vi "OdorSystem-counter-V1.vi"() -> ()   [LabVIEW 2019]
doc: "Synchronize Correlated Digital Output with Analog Input Using NI-DAQmx \n\nOverview:\nThis example uses DAQmx to synchronize finite generation and acquisition of Correlated Digital Output with an Analog Input Task respectively.\n\nDescriptions:\nCorrelated I/O enables synchronization of on board digital I/O lines to a clock reference. Digital and Analog samples can be synchronized in time by sharing the AI clock as the source of your digital I/O clock. You may also use the Counter Output pulse as the Source of Digital Timing. Hence, set the Source for Digital Timing as ai/SampleClock.This example will work on any device that uses DAQmx and supports Correlated Digital I/O. To perform Correlated Digital I/O on 9172 Chassis, you need a Correlated Module in slot 1-4 of the chassis. \n\nRequirements:\n1. LabVIEW 2012 or compatible.\n2. NI-DAQmx 15.5.1 or compatible.\n\nInstructions:\n1. Set all the control values on the front panel corresponding to the physical channel to be used on the DAQ device.\n2. Run this VI.\n3. Monitor the analog input voltage measured and ramp signal generated from specified channels. \n\nBlock Diagram Steps:\n1. Creates channels to measure voltage and to generate digital signals \n2. Sets the source of the Sample Clock, the rate of the Sample Clock, and the number of samples to acquire or generate.\n3. Generates an array containing a ramp pattern and write to digital output lines.\n4. Transitions the tasks to running state to begin measuring and generating data.\n5. Reads the waveform from the analog input channel and waits for the digital output generation to complete.\n6. Clears the tasks.\n7. Displays any error occurs."
uses:
  StatesEnum.ctl
  <vilib>/DAQmx/write.llb/DAQmx Write (Digital 1D Bool NChan 1Samp 1Line).vi
  <vilib>/DAQmx/write.llb/DAQmx Write (Digital Wfm 1Chan NSamp).vi
  <vilib>/DAQmx/miscellaneous.llb/DAQmx Fill In Error Info.vi
  <vilib>/DAQmx/create/channels.llb/DAQmx Create Channel (CO-Pulse Generation-Frequency).vi
  <vilib>/Waveform/DWDTOps.llb/Digital Pattern Generator (Single Value).vi
  <vilib>/Waveform/DWDTOps.llb/DWDT Append Digital Samples.vi
  <vilib>/DAQmx/configure/timing.llb/DAQmx Timing (Implicit).vi
  <vilib>/Waveform/DWDTOps.llb/DWDT Append Digital Signals.vi
  <vilib>/Waveform/DWDTOps.llb/DWDT Digital to Boolean Array.vi
  <vilib>/DAQmx/create/channels.llb/DAQmx Create Channel (DO-Digital Output).vi
  <vilib>/DAQmx/configure/timing.llb/DAQmx Timing (Sample Clock).vi
  <vilib>/Waveform/DWDTOps.llb/DWDT Uncompress Digital.vi
panel:
  out "Experiment running":bool
  out "State":T1
  in  "Select experiment":enum32{"Single trial", "Trial series"}(tab)
  out "Time elapsed":dbl format="%.1f"
  in  "Start single trial":bool
  out "single trial done":bool
  in  "Select valve":u8(knob)=1 min=1 max=8 step=1 scale=1.0..8.0
  out "Pause elapsed time":dbl format="%#.1f"
  out "In between trials":bool
  out "Trial elapsed time":dbl format="%.1f"
  out "Total elapsed time":dbl format="%.1f"
  out "Estimated total time":dbl
  out "Current list index":i32
  out "Current Valve":u8
  in  "Time between trials":u16=10 min=1 max=900 step=1
  in  "Start trial series":bool
  in  "Valve order list":i8[](array[numeric]) min=1 max=8 step=1
  out "Digitaler output":digitalwaveform(graph)
  out "Stop Boolesch":bool
  in  "Total trial time":dbl=20.0 min=1.0 step=0.1
  in  "Valve opening Time":dbl=10.0 min=0.0 step=0.1
  in  "Valve delay":dbl=2.0 min=0.0 step=0.1
  in  "Stopp":bool
  out "Digital Waveform Graph":digitalwaveform(graph)
  # "All times are in second!"
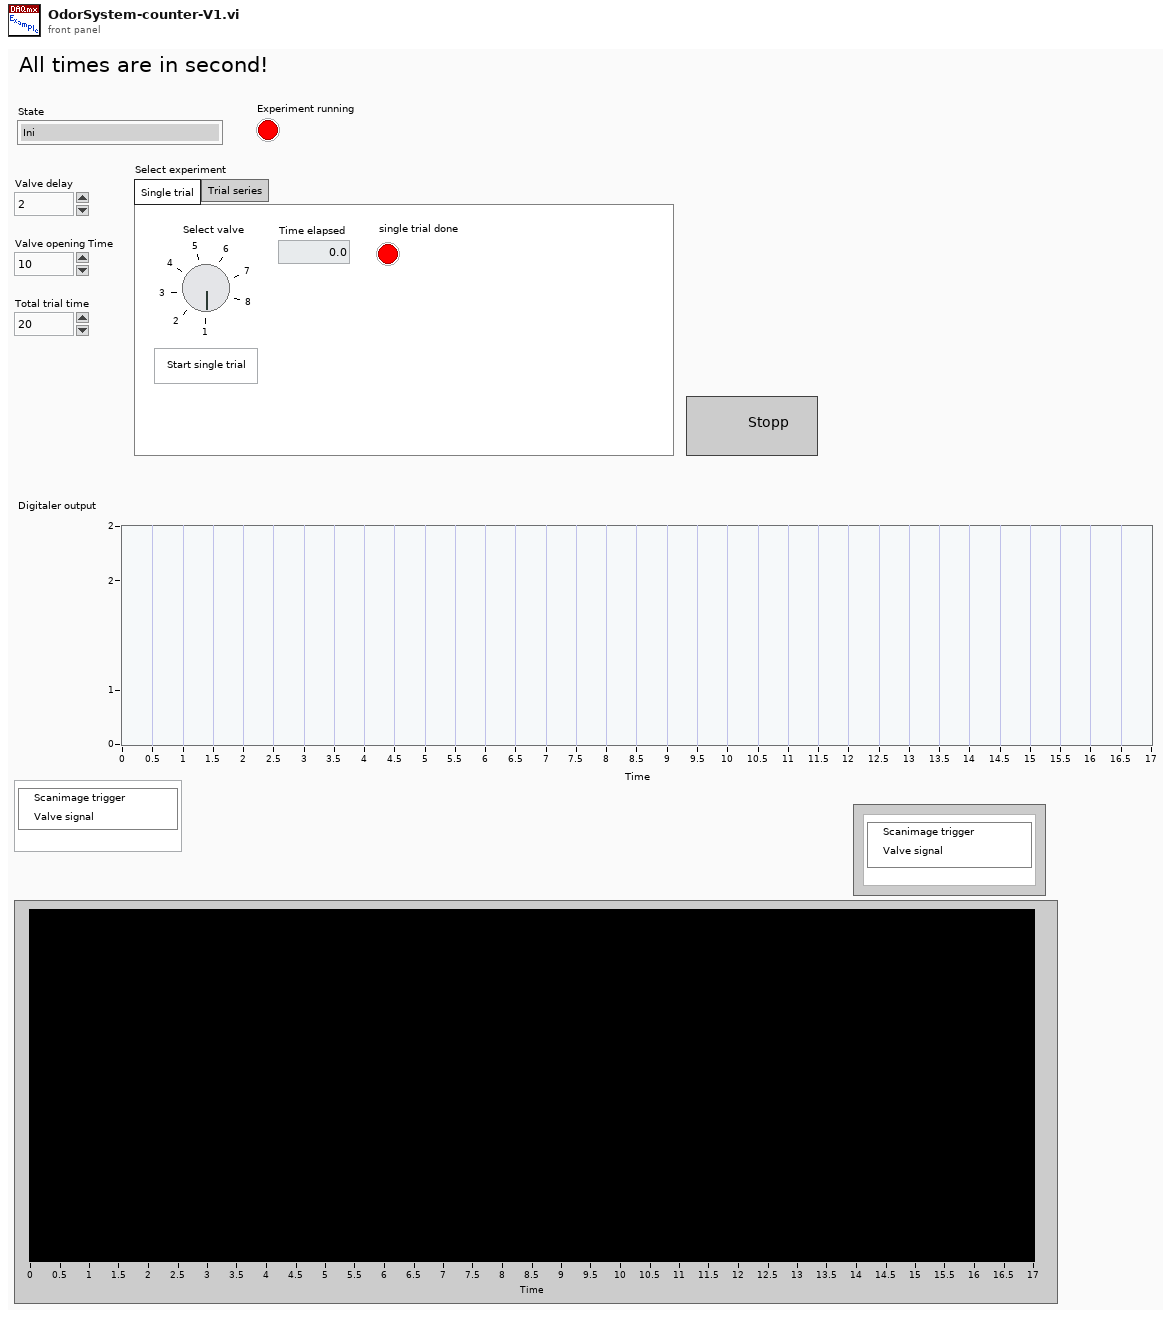
[diagram p1: front panel]
types:
  T1 = typedef "StatesEnum.ctl" = enum16{"Ini", "Standby", "Start Trial", "Start trial series", "Stop"}
  T2 = enum8{"Enabled", "Disabled", "Disabled and Grayed Out"}
  T3 = enum32{"Page Enabled", "Page Disabled", "Page Disabled & Grayed"}
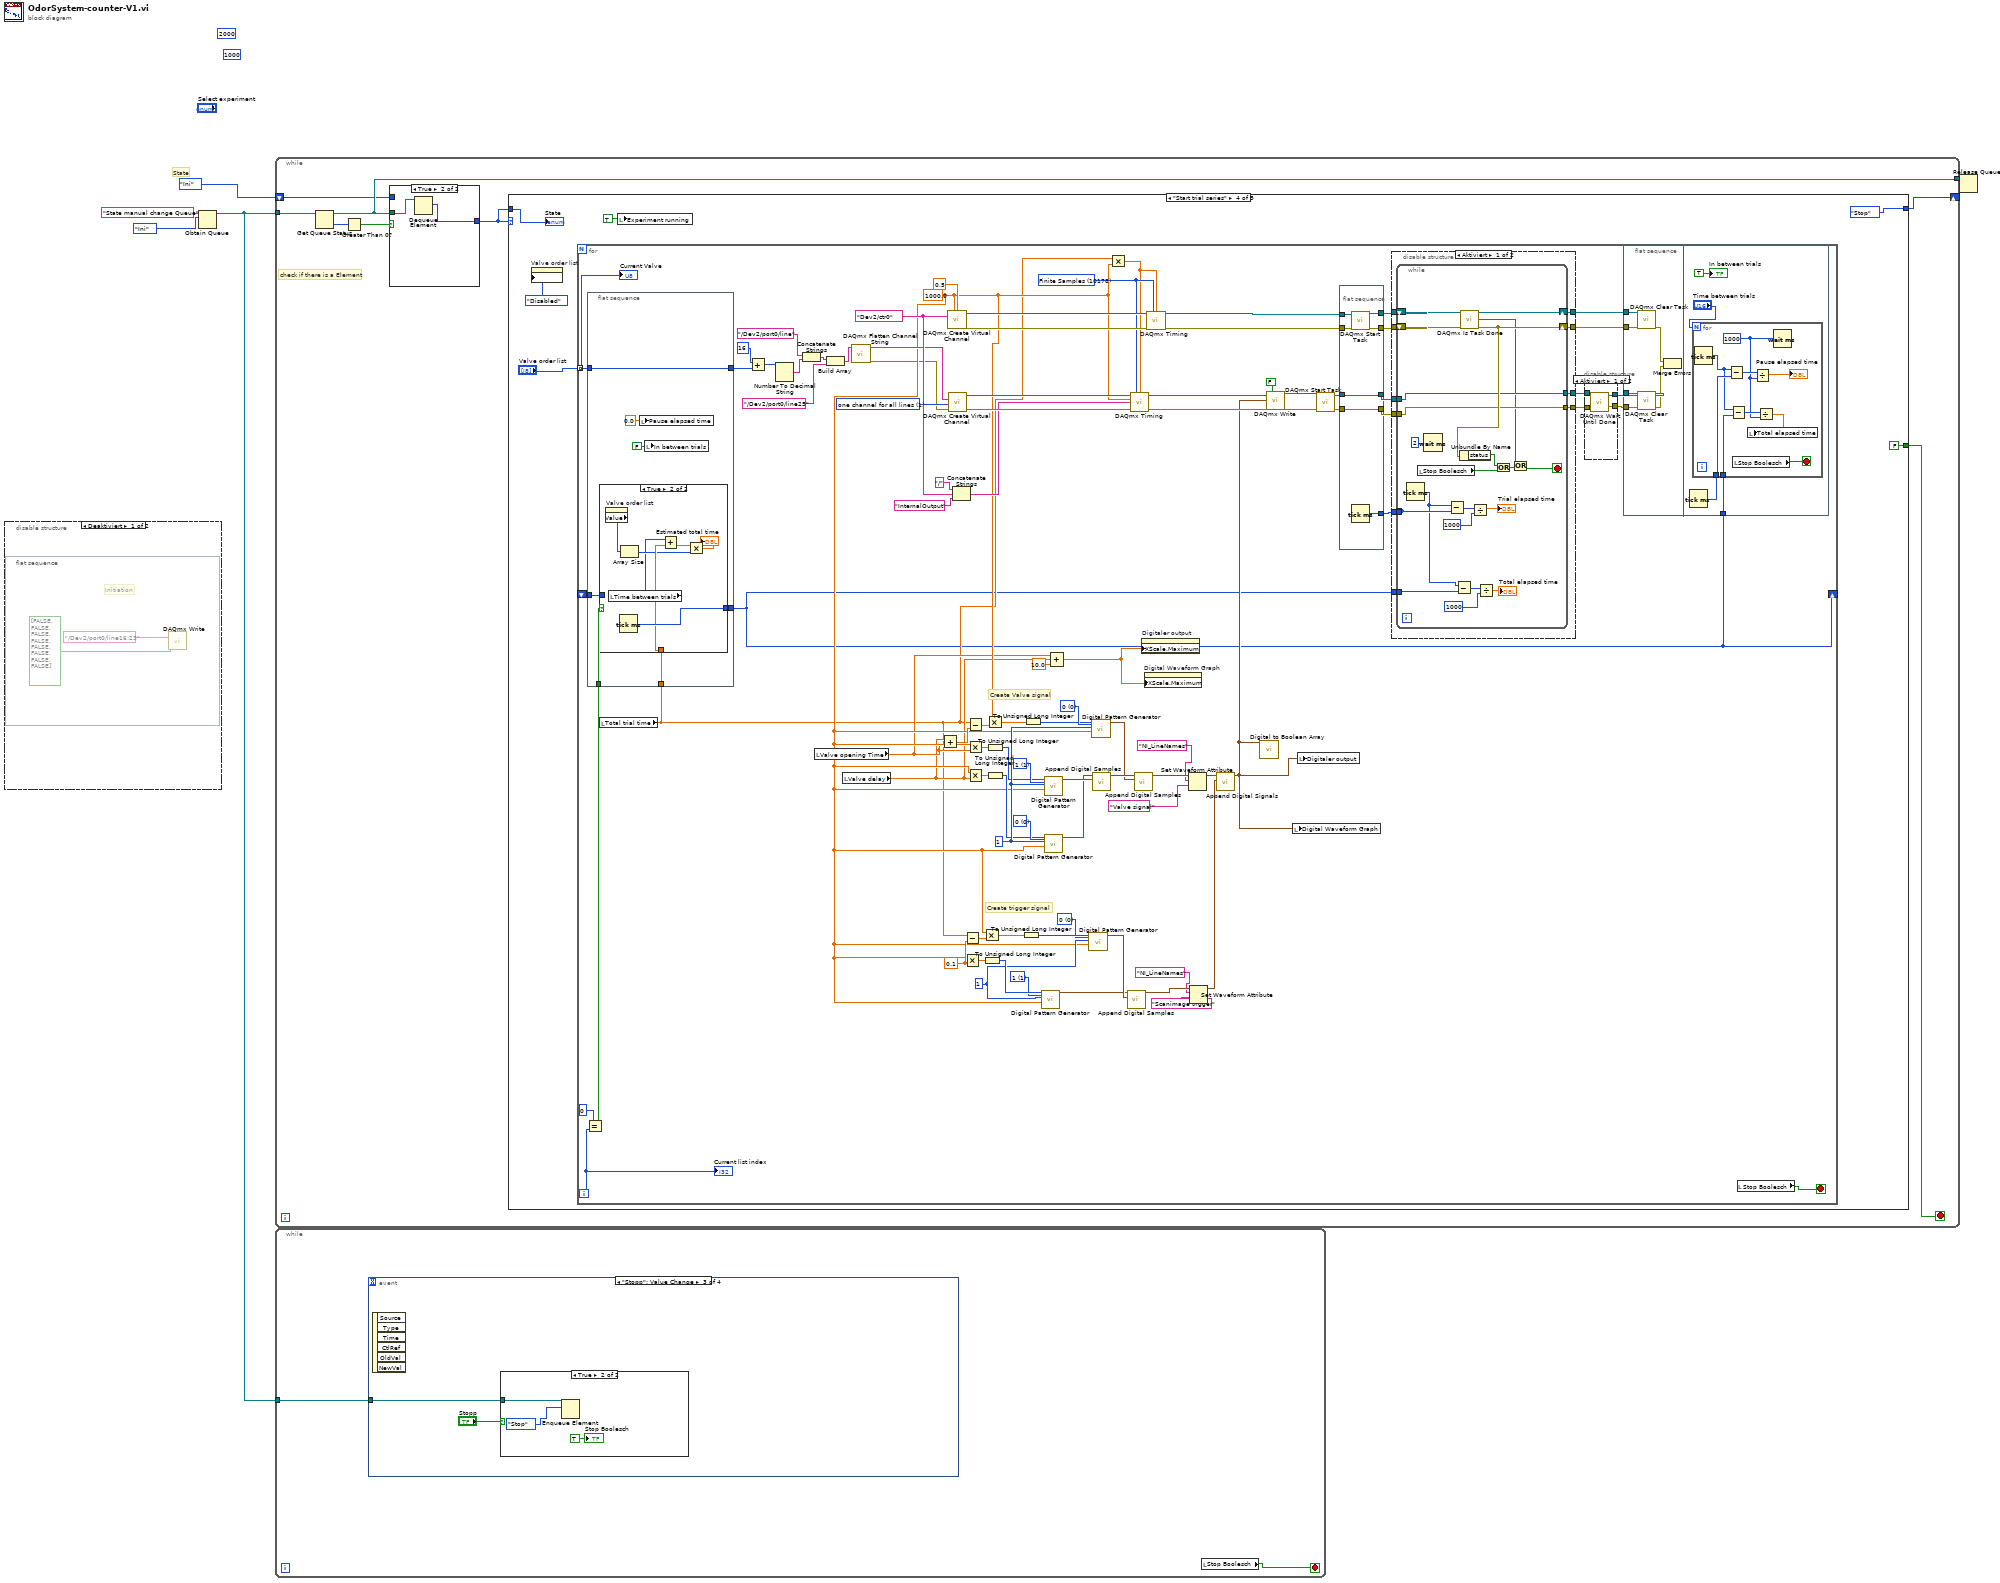
[diagram p0: block diagram]
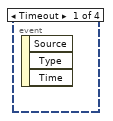
[diagram p3: hidden frame]
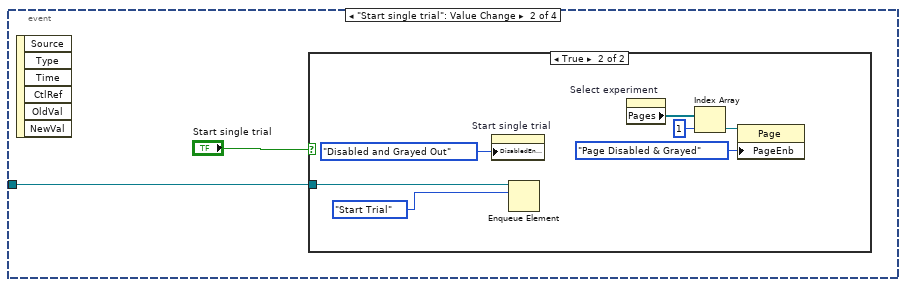
[diagram p4: hidden frame]
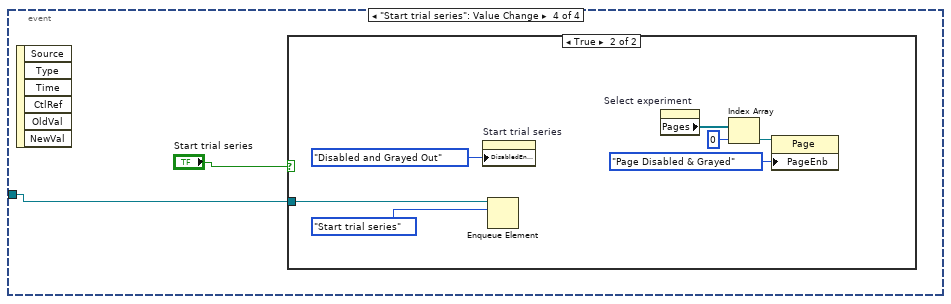
[diagram p7: hidden frame]
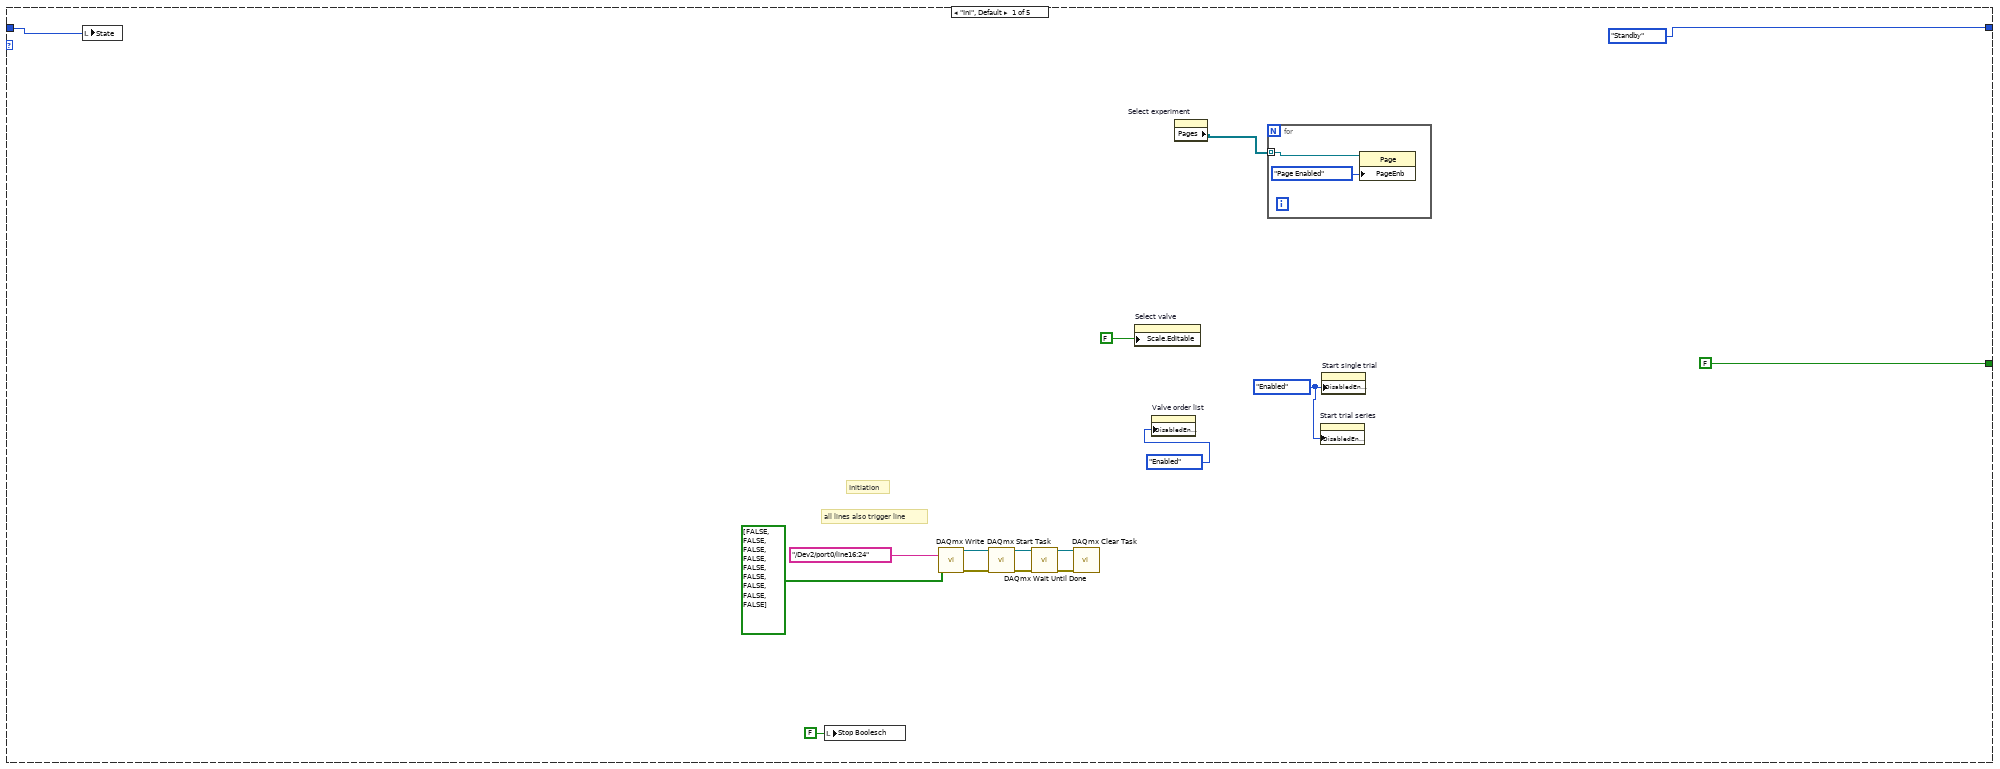
[diagram p10: hidden frame]
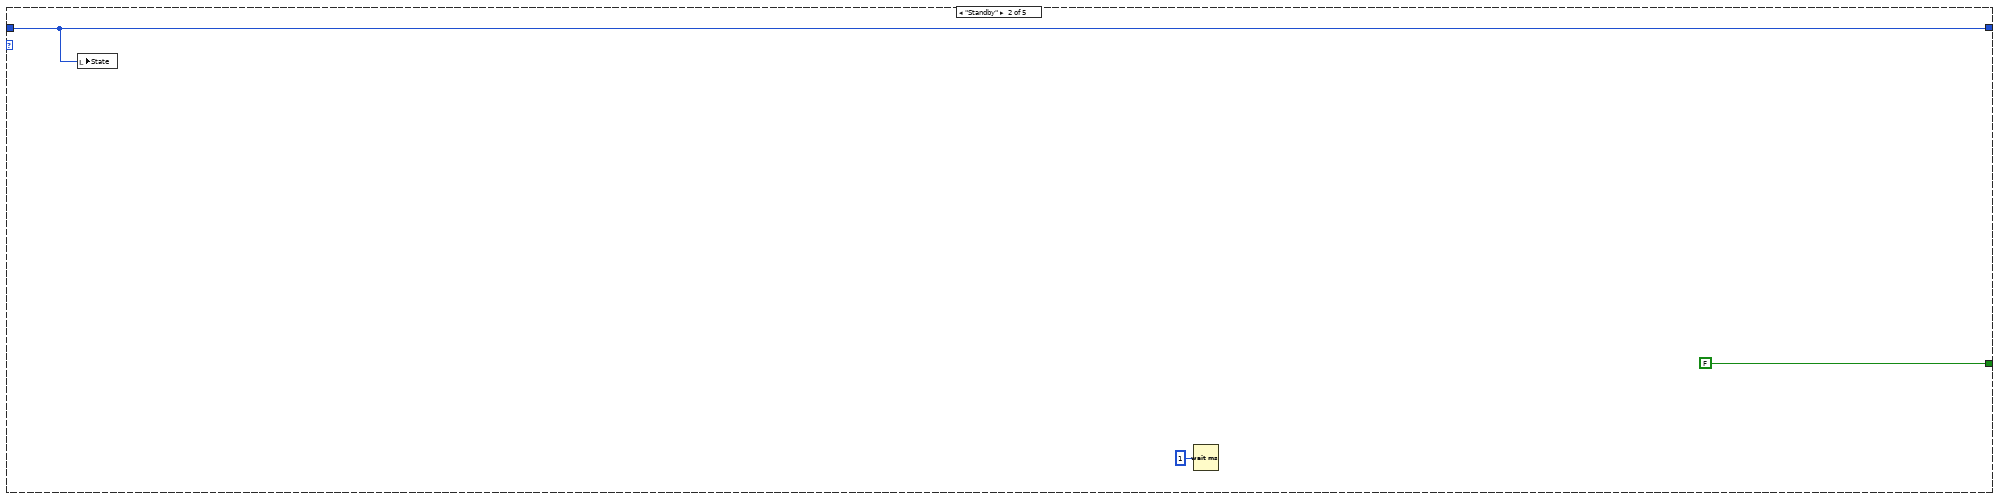
[diagram p11: hidden frame]
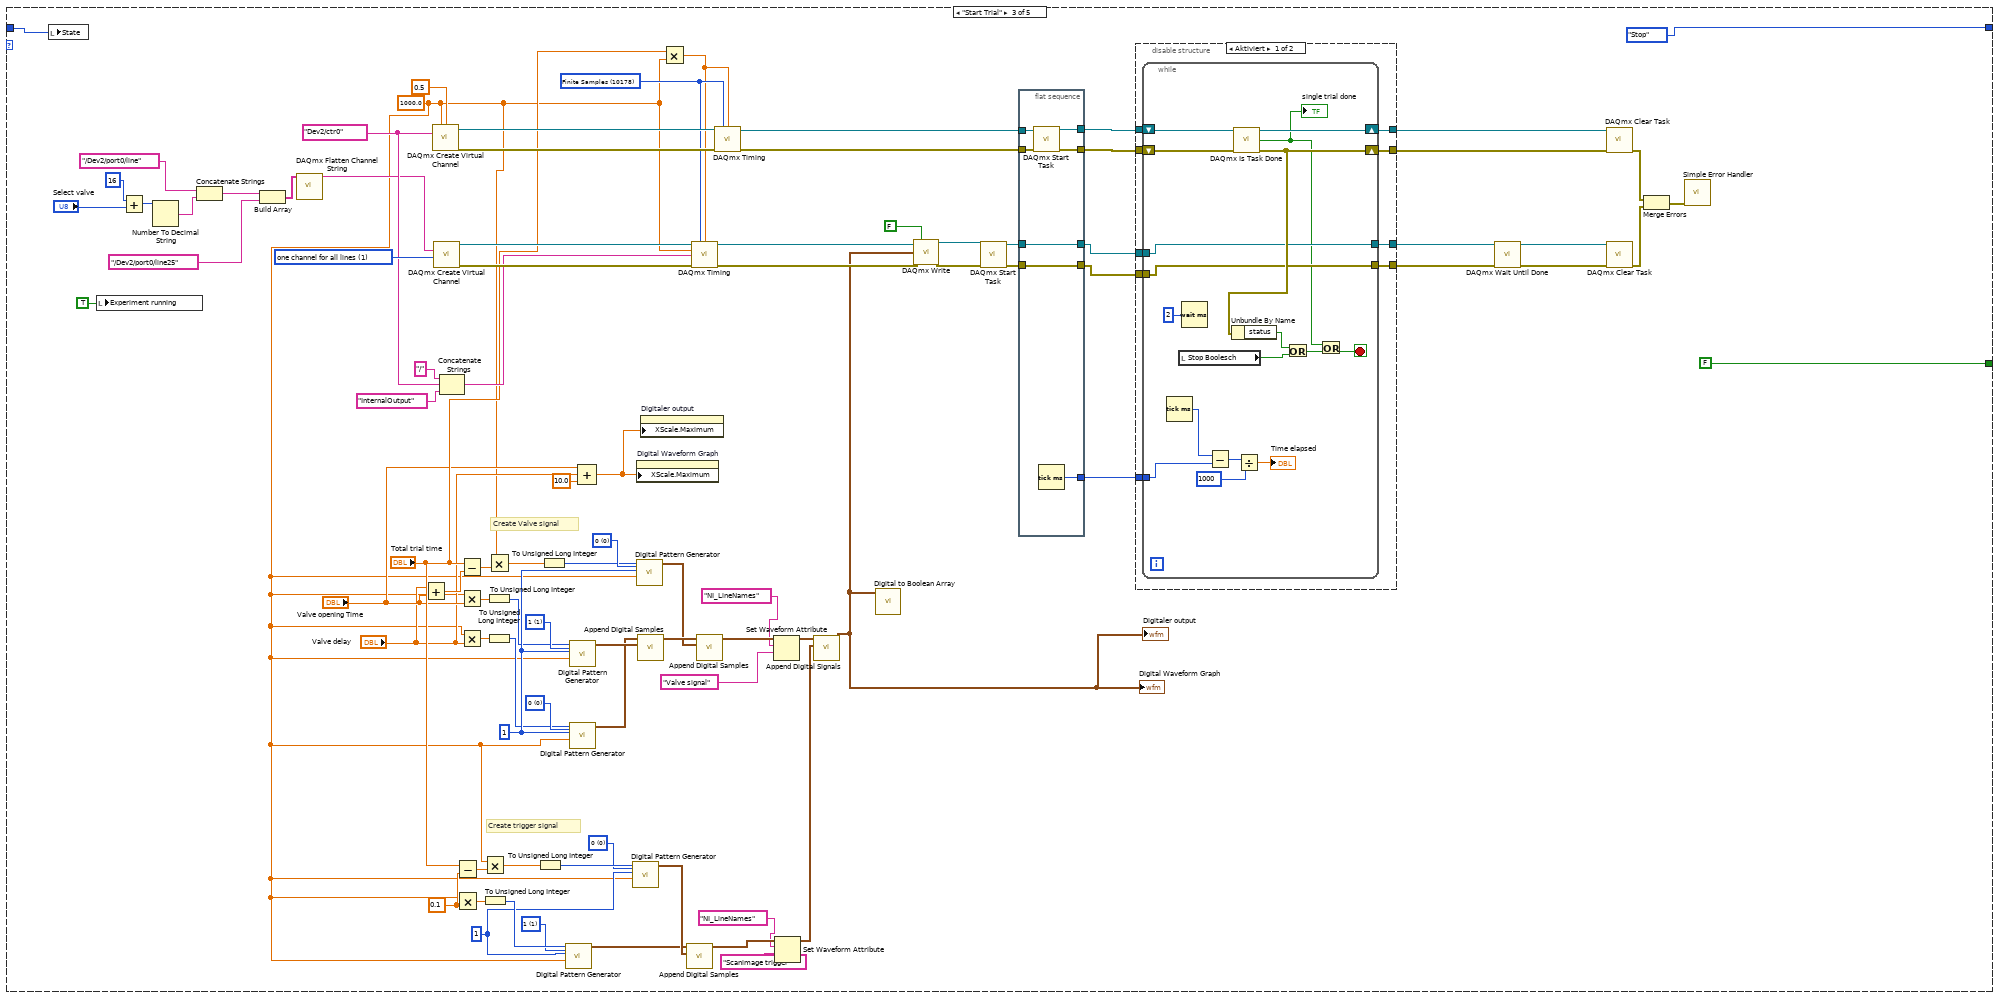
[diagram p12: hidden frame]
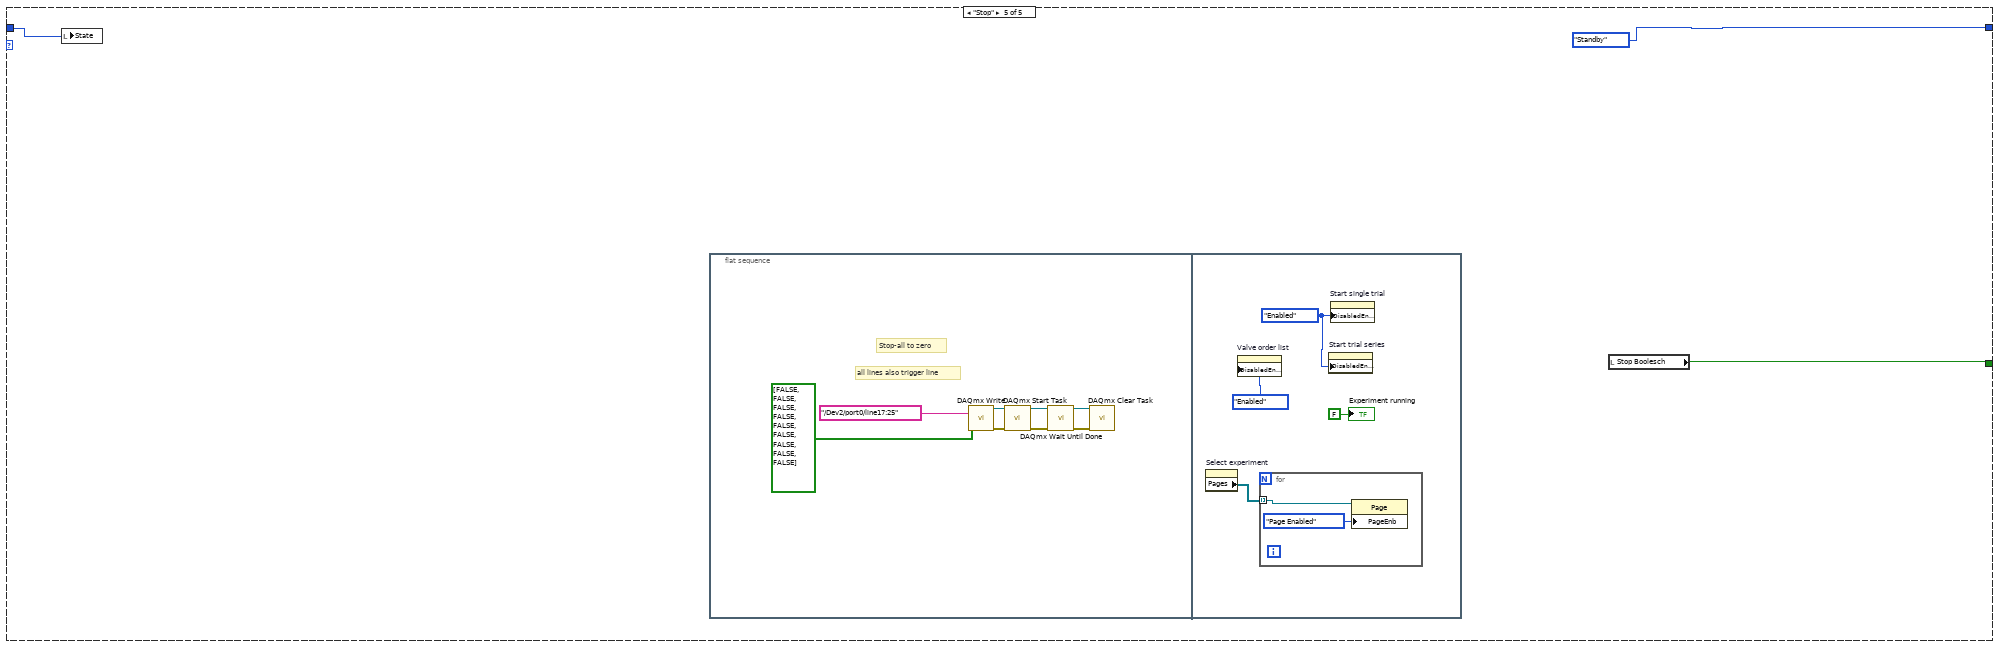
[diagram p17: hidden frame]
diagram:
  (unwired) u32 2000 ("number of samples")
  (unwired) u32 1000 ("number of samples")
  # "State"
  n1 = disable-structure shown="Deaktiviert" {
    frame Disabled {
      n2 = flat-sequence {
        frame #0 {
          # "Initiation"
          n3 = call-poly <vilib>:"DAQmx Write.vi"("task/channels in"="/Dev2/port0/line16:23" ("string"), "data"=bool[] [FALSE, FALSE, FALSE, FALSE, FALSE, FALSE, FALSE, FALSE]) -> ()  [unwired: 11 in, 3 out]
        }
      }
    }
    frame Enabled {
    }
  }
  n4 = Obtain Queue(name (unnamed)="State manual change Queue", element data type=StatesEnum."Ini" ("Enum")) -> (queue out=w4:refnum<queue>)  [unwired: 3 in, 2 out]
  n5 = while {
    tunnel: w4 -> [w13]
    tunnel: [w12] -> w3
    shift-right: [w8] -> _
    shift-left: StatesEnum."Ini" -> [w9]
    stop <- w11 stop-if-true
    # "check if there is a Element"
    n6 = Get Queue Status(queue=w13) -> (queue out=w12:refnum<queue>, # elements in queue=w15:i32)  [unwired: 2 in, 6 out]
    n7 = Greater Than 0?(x=w15) -> (x > 0?=w14:bool)
    n8 = case shown="True" w14 {
      tunnel: w12 -> [_ w18]
      tunnel: w9 -> [w16 _]
      tunnel: [w16 w17] -> w10
      frame False {
      }
      frame True {
        n9 = Dequeue Element(queue=w18) -> (element=w17:T1)  [unwired: 2 in, 3 out]
      }
    }
    n10 = case shown="\"Start trial series\"" w10 {
      tunnel: w10 -> [w29 w37 w43 w165 w335]
      tunnel: [FALSE ("Stop Boolesch") FALSE ("Stop Boolesch") FALSE ("Stop Boolesch") FALSE ("Stop Boolesch") w337] -> w11
      tunnel: [StatesEnum."Standby" ("Enum") w37 StatesEnum."Stop" ("Enum") StatesEnum."Stop" ("Enum") StatesEnum."Standby" ("Enum")] -> w8
      frame "Ini", Default {
        w22 = T2."Enabled" ("Deaktiviert")
        # "all lines also trigger line"
        # "Initiation"
        n11 = local write "State"(w29) -> ()
        n12 = local write "Stop Boolesch"(FALSE ("Stop Boolesch")) -> ()
        n13 = call-poly <vilib>:"DAQmx Write.vi"("task/channels in"="/Dev2/port0/line16:24" ("string"), "data"=bool[] [FALSE, FALSE, FALSE, FALSE, FALSE, FALSE, FALSE, FALSE, FALSE]) -> ("task out"=w24:refnum<k21>, "error out"=w23:errorcluster)  [unwired: 11 in, 1 out]
        n14 = call <vilib>:"DAQmx Start Task.vi"("task/channels in"=w24, "error in"=w23) -> ("task out"=w28:refnum<k21>, "error out"=w26:errorcluster)  [unwired: 12 in]
        n15 = call <vilib>:"DAQmx Wait Until Done.vi"("task/channels in"=w28, "error in"=w26) -> ("task out"=w27:refnum<k21>, "error out"=w25:errorcluster)  [unwired: 12 in]
        n16 = call <vilib>:"DAQmx Clear Task.vi"("task in"=w27, "error in"=w25) -> ()  [unwired: 13 in, 1 out]
        n17 = property on="Select valve" class="Knob (strict)"("Scale.Editable"=FALSE ("Skala.Editierbar")) -> ()  [unwired: 2 in, 2 out]
        n18 = property on="Valve order list" class="Arr (strict)"("DisabledEnum"=T2."Enabled" ("Deaktiviert")) -> ()  [unwired: 2 in, 2 out]
        n19 = property on="Select experiment" class="TabCtl (strict)"() -> ("Pages"=w20:refnum<vi>[])  [unwired: 2 in, 2 out]
        n20 = for {
          tunnel: w20 -> [w35] mode=indexing
          n21 = property class="Page"(reference=w35, "PageEnb"=T3."Page Enabled" ("Aktiv-Status der Seite")) -> ()  [unwired: 1 in, 2 out]
        }
        n22 = property on="Start trial series" class="Bool"("DisabledEnum"=w22) -> ()  [unwired: 2 in, 2 out]
        n23 = property on="Start single trial" class="Bool"("DisabledEnum"=w22) -> ()  [unwired: 2 in, 2 out]
      }
      frame "Standby" {
        n24 = local write "State"(w37) -> ()
        n25 = Wait (ms)(milliseconds to wait=u32 1 ("Zu wartende ms")) -> ()  [unwired: 1 out]
      }
      frame "Start Trial" {
        w67 = 0.1 ("y")
        w74 = u32 1 ("number of signals")
        w76 = u8 0 items=["0", "1", "Z", "L", "H", "X", "T", "V"] ("value")
        w75 = u8 1 items=["0", "1", "Z", "L", "H", "X", "T", "V"] ("value")
        w95 = tag "Dev2/ctr0" ("counter")
        w49 = 1000.0 ("frequency")
        w104 = u32 1 ("number of signals")
        w105 = u8 0 items=["0", "1", "Z", "L", "H", "X", "T", "V"] ("value")
        w106 = u8 1 items=["0", "1", "Z", "L", "H", "X", "T", "V"] ("value")
        w107 = u8 0 items=["0", "1", "Z", "L", "H", "X", "T", "V"] ("value")
        w118 = 1 items=["one channel for each line", "one channel for all lines"] ("line grouping")
        w99 = 10178 items=["Finite Samples"=10178, "Continuous Samples"=10123] ("sample mode")
        # "Create trigger signal"
        # "Create Valve signal"
        n26 = local write "State"(w43) -> ()
        n27 = local write "Experiment running"(TRUE ("Experiment running")) -> ()
        n28 = Add(x=i8 16, y="Select valve") -> (x+y=w83:u8)
        n29 = Number To Decimal String(number=w83) -> (decimal integer string=w84:string)  [unwired: 1 in]
        n30 = Concatenate Strings("/Dev2/port0/line" ("string"), w84) -> (w73:string)
        n31 = Build Array(w73, "/Dev2/port0/line25" ("string")) -> (w71:string[])
        n32 = call <vilib>:"DAQmx Flatten Channel String.vi"("names in"=w71) -> ("names out"=w70:string)  [unwired: 13 in, 1 out]
        n33 = Add(x="Valve delay", y="Valve opening Time") -> (x+y=w87:dbl)
        n34 = call-poly <vilib>:"DAQmx Create Virtual Channel.vi"("frequency"=w49, "duty cycle"=0.5, "counter"=w95) -> ("task out"=w123:refnum<k21>, "error out"=w124:errorcluster)  [unwired: 11 in]
        n35 = call-poly <vilib>:"DAQmx Create Virtual Channel.vi"("lines"=w70, "line grouping"=w118) -> ("task out"=w128:refnum<k21>, "error out"=w127:errorcluster)  [unwired: 12 in]
        n36 = Concatenate Strings("/", w95, "InternalOutput" ("string")) -> (w94:string)
        n37 = Subtract(x="Total trial time", y=w67) -> (x-y=w81:dbl)
        n38 = Multiply(x=w49, y=w67) -> (x*y=w77:dbl)
        n39 = Subtract(x="Total trial time", y=w87) -> (x-y=w86:dbl)
        n40 = Multiply(x=w49, y="Valve opening Time") -> (x*y=w91:dbl)
        n41 = Multiply(x=w49, y="Valve delay") -> (x*y=w93:dbl)
        n42 = Multiply(x=w49, y=w81) -> (x*y=w79:dbl)
        n43 = To Unsigned Long Integer(number=w77) -> (unsigned 32bit integer=w78:u32)
        n44 = Multiply(x=w49, y=w86) -> (x*y=w89:dbl)
        n45 = To Unsigned Long Integer(number=w91) -> (unsigned 32bit integer=w90:u32)
        n46 = To Unsigned Long Integer(number=w93) -> (unsigned 32bit integer=w92:u32)
        n47 = To Unsigned Long Integer(number=w79) -> (unsigned 32bit integer=w80:u32)
        n48 = To Unsigned Long Integer(number=w89) -> (unsigned 32bit integer=w88:u32)
        n49 = call-poly <vilib>:"Digital Pattern Generator.vi"("value"=w75, "sample rate"=w49, "number of signals"=w74, "number of samples"=w78) -> ("digital waveform"=w55:digitalwaveform)  [unwired: 6 in, 1 out]
        n50 = call-poly <vilib>:"Digital Pattern Generator.vi"("value"=w106, "sample rate"=w49, "number of signals"=w104, "number of samples"=w90) -> ("digital waveform"=w60:digitalwaveform)  [unwired: 6 in, 1 out]
        n51 = call-poly <vilib>:"Digital Pattern Generator.vi"("value"=w107, "sample rate"=w49, "number of signals"=w104, "number of samples"=w92) -> ("digital waveform"=w59:digitalwaveform)  [unwired: 6 in, 1 out]
        n52 = Compound Arithmetic op=ADD("Valve opening Time", "Valve delay", 10.0 ("Wert")) -> (w44:dbl)
        n53 = call-poly <vilib>:"Digital Pattern Generator.vi"("value"=w76, "sample rate"=w49, "number of signals"=w74, "number of samples"=w80) -> ("digital waveform"=w56:digitalwaveform)  [unwired: 6 in, 1 out]
        n54 = property on="Digital Waveform Graph" class="DigitalGraph (strict)"("XScale.Maximum"=w44) -> ()  [unwired: 2 in, 2 out]
        n55 = call-poly <vilib>:"Digital Pattern Generator.vi"("value"=w105, "sample rate"=w49, "number of signals"=w104, "number of samples"=w88) -> ("digital waveform"=w57:digitalwaveform)  [unwired: 6 in, 1 out]
        n56 = call-poly <vilib>:"Append Digital Samples.vi"("digital waveform B"=w60, "digital waveform A"=w59) -> ("digital waveform out"=w58:digitalwaveform)  [unwired: 8 in, 1 out]
        n57 = property on="Digitaler output" class="DigitalGraph (strict)"("XScale.Maximum"=w44) -> ()  [unwired: 2 in, 2 out]
        n58 = Multiply(x="Total trial time", y=w49) -> (x*y=w68:dbl)
        n59 = call-poly <vilib>:"Append Digital Samples.vi"("digital waveform B"=w56, "digital waveform A"=w55) -> ("digital waveform out"=w66:digitalwaveform)  [unwired: 8 in, 1 out]
        n60 = call-poly <vilib>:"DAQmx Timing.vi"("task/channels in"=w128, "sample mode"=w99, "samples per channel"=w68, "rate"=w49, "source"=w94, "error in"=w127) -> ("task out"=w115:refnum<k21>, "error out"=w114:errorcluster)  [unwired: 8 in]
        n61 = call-poly <vilib>:"Append Digital Samples.vi"("digital waveform B"=w57, "digital waveform A"=w58) -> ("digital waveform out"=w63:digitalwaveform)  [unwired: 8 in, 1 out]
        n62 = call-poly <vilib>:"DAQmx Timing.vi"("task/channels in"=w123, "sample mode"=w99, "samples per channel"=w68, "error in"=w124) -> ("task out"=w121:refnum<k21>, "error out"=w122:errorcluster)  [unwired: 10 in]
        n63 = Set Waveform Attribute(5:"Valve signal", 6:"NI_LineNames" ("name"), 7:w63) -> (3:w54:digitalwaveform)  [unwired: 1 in, 2 out]
        n64 = Set Waveform Attribute(5:"Scanimage trigger", 6:"NI_LineNames" ("name"), 7:w66) -> (3:w53:digitalwaveform)  [unwired: 1 in, 2 out]
        n65 = call-poly <vilib>:"Append Digital Signals.vi"("digital waveform (low bits)"=w53, "digital waveform (high bits)"=w54) -> ("digital waveform out"=w46:digitalwaveform)  [unwired: 8 in, 1 out]
        "Digital Waveform Graph" <- w46
        "Digitaler output" <- w46
        n66 = call-poly <vilib>:"Digital to Boolean Array.vi"("digital waveform"=w46) -> ()  [unwired: 9 in, 2 out]
        n67 = call-poly <vilib>:"DAQmx Write.vi"("task/channels in"=w115, "auto start"=FALSE, "data"=w46, "error in"=w114) -> ("task out"=w113:refnum<k21>, "error out"=w112:errorcluster)  [unwired: 9 in, 1 out]
        n68 = call <vilib>:"DAQmx Start Task.vi"("task/channels in"=w113, "error in"=w112) -> ("task out"=w117:refnum<k21>, "error out"=w116:errorcluster)  [unwired: 12 in]
        n69 = flat-sequence {
          tunnel: [w161] -> w126
          tunnel: [w160] -> w125
          tunnel: w122 -> [w159]
          tunnel: w121 -> [w158]
          tunnel: [w157] -> w103
          tunnel: w117 -> [w157]
          tunnel: [w156] -> w102
          tunnel: w116 -> [w156]
          tunnel: [w155] -> w41
          frame #0 {
            n70 = call <vilib>:"DAQmx Start Task.vi"("task/channels in"=w158, "error in"=w159) -> ("task out"=w161:refnum<k21>, "error out"=w160:errorcluster)  [unwired: 12 in]
            n71 = Tick Count (ms)() -> (millisecond timer value=w155:u32)
          }
        }
        n72 = disable-structure shown="Aktiviert" {
          disable-tunnel: w126 -> [w137 _]
          disable-tunnel: w125 -> [w136 _]
          disable-tunnel: [w135 _] -> w120
          disable-tunnel: [w134 _] -> w119
          disable-tunnel: w103 -> [w133 _]
          disable-tunnel: w102 -> [w132 _]
          disable-tunnel: [w131 _] -> w101
          disable-tunnel: [w130 _] -> w100
          disable-tunnel: w41 -> [w129 _]
          frame Enabled {
            n73 = while {
              shift-right: [w151] -> w134
              shift-left: w137 -> [w153]
              shift-right: [w150] -> w135
              shift-left: w136 -> [w152]
              tunnel: w133 -> [w149]
              tunnel: w132 -> [w148]
              tunnel: [w149] -> w131
              tunnel: [w148] -> w130
              tunnel: w129 -> [w141]
              stop <- w144 stop-if-true
              n74 = Tick Count (ms)() -> (millisecond timer value=w142:u32)
              n75 = local read "Stop Boolesch"() -> (w145:bool)
              n76 = Wait (ms)(milliseconds to wait=u32 2 ("Zu wartende ms")) -> ()  [unwired: 1 out]
              n77 = Subtract(x=w142, y=w141) -> (x-y=w140:u32)
              n78 = call <vilib>:"DAQmx Is Task Done.vi"("task/channels in"=w153, "error in"=w152) -> ("task out"=w151:refnum<k21>, "task done?"=w143:bool, "error out"=w150:errorcluster)  [unwired: 11 in]
              "single trial done" <- w143
              n79 = Unbundle By Name(w150) -> ("status"=w146:bool)
              n80 = Divide(x=w140, y=u32 1000) -> (x/y=→"Time elapsed":dbl)
              n81 = Or(x=w146, y=w145) -> (x .or. y?=w154:bool)
              n82 = Or(x=w143, y=w154) -> (x .or. y?=w144:bool)
            }
          }
          frame Disabled {
          }
        }
        n83 = call <vilib>:"DAQmx Wait Until Done.vi"("task/channels in"=w101) -> ("task out"=w48:refnum<k21>)  [unwired: 13 in, 1 out]
        n84 = call <vilib>:"DAQmx Clear Task.vi"("task in"=w119, "error in"=w120) -> ("error out"=w110:errorcluster)  [unwired: 13 in]
        n85 = call <vilib>:"DAQmx Clear Task.vi"("task in"=w48, "error in"=w100) -> ("error out"=w109:errorcluster)  [unwired: 13 in]
        n86 = Merge Errors(w110, w109) -> (w108:errorcluster)
        n87 = call <vilib>:"Simple Error Handler.vi"("error in (no error)"=w108) -> ()  [unwired: 4 in, 5 out]
      }
      frame "Start trial series" {
        n88 = property on="Valve order list" class="Arr (strict)"("DisabledEnum"=T2."Disabled" ("Deaktiviert")) -> ()  [unwired: 2 in, 2 out]
        n89 = for {
          tunnel: "Valve order list" -> [w173] mode=indexing
          shift-right: [w169] -> _
          shift-left: _ -> [w171]
          i -> [w179]
          stop <- w183 stop-if-true
          w204 = 0.1 ("y")
          w210 = u32 1 ("number of signals")
          w212 = u8 0 items=["0", "1", "Z", "L", "H", "X", "T", "V"] ("value")
          w211 = u8 1 items=["0", "1", "Z", "L", "H", "X", "T", "V"] ("value")
          w231 = tag "Dev2/ctr0" ("counter")
          w188 = 1000.0 ("frequency")
          w239 = u32 1 ("number of signals")
          w240 = u8 0 items=["0", "1", "Z", "L", "H", "X", "T", "V"] ("value")
          w241 = u8 1 items=["0", "1", "Z", "L", "H", "X", "T", "V"] ("value")
          w242 = u8 0 items=["0", "1", "Z", "L", "H", "X", "T", "V"] ("value")
          w250 = 1 items=["one channel for each line", "one channel for all lines"] ("line grouping")
          w235 = 10178 items=["Finite Samples"=10178, "Continuous Samples"=10123] ("sample mode")
          # "Create trigger signal"
          # "Create Valve signal"
          n90 = Equal?(x=0, y=w179) -> (x = y?=w172:bool)
          n91 = flat-sequence {
            tunnel: [w269] -> w174
            tunnel: w173 -> [w269]
            tunnel: w172 -> [w268]
            tunnel: w171 -> [w267]
            tunnel: w170 -> [w266]
            tunnel: [w265] -> w169
            frame #0 {
              n92 = case shown="True" w268 {
                tunnel: [w270 w277] -> w265
                tunnel: w267 -> [w270 _]
                tunnel: w266 -> [_ w276]
                frame False {
                }
                frame True {
                  n93 = property on="Valve order list" class="Arr (strict)"() -> ("Value"=w274:i8[])  [unwired: 2 in, 2 out]
                  n94 = local read "Time between trials"() -> (w271:u16)
                  n95 = Tick Count (ms)() -> (millisecond timer value=w277:u32)
                  n96 = Array Size(array=w274) -> (size(s)=w273:i32)
                  n97 = Add(x=w271, y=w276) -> (x+y=w272:dbl)
                  n98 = Multiply(x=w272, y=w273) -> (x*y=→"Estimated total time":dbl)
                }
              }
              n99 = local write "Pause elapsed time"(0.0 ("Pause elapsed time")) -> ()
              n100 = local write "In between trials"(FALSE ("In between trials")) -> ()
            }
          }
          n101 = local read "Total trial time"() -> (w170:dbl)
          n102 = Add(x=i8 16, y=w174) -> (x+y=w219:i8)
          n103 = Number To Decimal String(number=w219) -> (decimal integer string=w220:string)  [unwired: 1 in]
          n104 = Concatenate Strings("/Dev2/port0/line" ("string"), w220) -> (w209:string)
          n105 = local read "Valve opening Time"() -> (w185:dbl)
          n106 = Build Array(w209, "/Dev2/port0/line25" ("string")) -> (w207:string[])
          n107 = local read "Valve delay"() -> (w184:dbl)
          n108 = call <vilib>:"DAQmx Flatten Channel String.vi"("names in"=w207) -> ("names out"=w206:string, "error out"=w168:errorcluster)  [unwired: 13 in]
          n109 = Add(x=w184, y=w185) -> (x+y=w223:dbl)
          n110 = call-poly <vilib>:"DAQmx Create Virtual Channel.vi"("frequency"=w188, "duty cycle"=0.5, "counter"=w231) -> ("task out"=w253:refnum<k21>, "error out"=w254:errorcluster)  [unwired: 11 in]
          n111 = call-poly <vilib>:"DAQmx Create Virtual Channel.vi"("lines"=w206, "line grouping"=w250, "error in"=w168) -> ("task out"=w258:refnum<k21>, "error out"=w257:errorcluster)  [unwired: 11 in]
          n112 = Concatenate Strings("/", w231, "InternalOutput" ("string")) -> (w230:string)
          n113 = Subtract(x=w170, y=w204) -> (x-y=w217:dbl)
          n114 = Multiply(x=w188, y=w204) -> (x*y=w213:dbl)
          n115 = Subtract(x=w170, y=w223) -> (x-y=w222:dbl)
          n116 = Multiply(x=w188, y=w185) -> (x*y=w227:dbl)
          n117 = Multiply(x=w188, y=w184) -> (x*y=w229:dbl)
          n118 = Multiply(x=w188, y=w217) -> (x*y=w215:dbl)
          n119 = To Unsigned Long Integer(number=w213) -> (unsigned 32bit integer=w214:u32)
          n120 = Multiply(x=w188, y=w222) -> (x*y=w225:dbl)
          n121 = To Unsigned Long Integer(number=w227) -> (unsigned 32bit integer=w226:u32)
          n122 = To Unsigned Long Integer(number=w229) -> (unsigned 32bit integer=w228:u32)
          n123 = To Unsigned Long Integer(number=w215) -> (unsigned 32bit integer=w216:u32)
          n124 = To Unsigned Long Integer(number=w225) -> (unsigned 32bit integer=w224:u32)
          n125 = call-poly <vilib>:"Digital Pattern Generator.vi"("value"=w211, "sample rate"=w188, "number of signals"=w210, "number of samples"=w214) -> ("digital waveform"=w192:digitalwaveform)  [unwired: 6 in, 1 out]
          n126 = call-poly <vilib>:"Digital Pattern Generator.vi"("value"=w241, "sample rate"=w188, "number of signals"=w239, "number of samples"=w226) -> ("digital waveform"=w197:digitalwaveform)  [unwired: 6 in, 1 out]
          n127 = call-poly <vilib>:"Digital Pattern Generator.vi"("value"=w242, "sample rate"=w188, "number of signals"=w239, "number of samples"=w228) -> ("digital waveform"=w196:digitalwaveform)  [unwired: 6 in, 1 out]
          n128 = Compound Arithmetic op=ADD(w185, w184, 10.0 ("Wert")) -> (w186:dbl)
          n129 = call-poly <vilib>:"Digital Pattern Generator.vi"("value"=w212, "sample rate"=w188, "number of signals"=w210, "number of samples"=w216) -> ("digital waveform"=w193:digitalwaveform)  [unwired: 6 in, 1 out]
          n130 = call-poly <vilib>:"Digital Pattern Generator.vi"("value"=w240, "sample rate"=w188, "number of signals"=w239, "number of samples"=w224) -> ("digital waveform"=w194:digitalwaveform)  [unwired: 6 in, 1 out]
          n131 = call-poly <vilib>:"Append Digital Samples.vi"("digital waveform B"=w197, "digital waveform A"=w196) -> ("digital waveform out"=w195:digitalwaveform)  [unwired: 8 in, 1 out]
          n132 = Multiply(x=w170, y=w188) -> (x*y=w205:dbl)
          n133 = call-poly <vilib>:"Append Digital Samples.vi"("digital waveform B"=w193, "digital waveform A"=w192) -> ("digital waveform out"=w203:digitalwaveform)  [unwired: 8 in, 1 out]
          n134 = call-poly <vilib>:"DAQmx Timing.vi"("task/channels in"=w258, "sample mode"=w235, "samples per channel"=w205, "rate"=w188, "source"=w230, "error in"=w257) -> ("task out"=w247:refnum<k21>, "error out"=w246:errorcluster)  [unwired: 8 in]
          n135 = call-poly <vilib>:"Append Digital Samples.vi"("digital waveform B"=w194, "digital waveform A"=w195) -> ("digital waveform out"=w200:digitalwaveform)  [unwired: 8 in, 1 out]
          n136 = property on="Digitaler output" class="DigitalGraph (strict)"("XScale.Maximum"=w186) -> ()  [unwired: 2 in, 2 out]
          n137 = property on="Digital Waveform Graph" class="DigitalGraph (strict)"("XScale.Maximum"=w186) -> ()  [unwired: 2 in, 2 out]
          n138 = call-poly <vilib>:"DAQmx Timing.vi"("task/channels in"=w253, "sample mode"=w235, "samples per channel"=w205, "error in"=w254) -> ("task out"=w251:refnum<k21>, "error out"=w252:errorcluster)  [unwired: 10 in]
          n139 = Set Waveform Attribute(5:"Valve signal", 6:"NI_LineNames" ("name"), 7:w200) -> (3:w191:digitalwaveform)  [unwired: 1 in, 2 out]
          n140 = Set Waveform Attribute(5:"Scanimage trigger", 6:"NI_LineNames" ("name"), 7:w203) -> (3:w190:digitalwaveform)  [unwired: 1 in, 2 out]
          n141 = call-poly <vilib>:"Append Digital Signals.vi"("digital waveform (low bits)"=w190, "digital waveform (high bits)"=w191) -> ("digital waveform out"=w187:digitalwaveform)  [unwired: 8 in, 1 out]
          n142 = call-poly <vilib>:"Digital to Boolean Array.vi"("digital waveform"=w187) -> ()  [unwired: 9 in, 2 out]
          n143 = call-poly <vilib>:"DAQmx Write.vi"("task/channels in"=w247, "auto start"=FALSE, "data"=w187, "error in"=w246) -> ("task out"=w245:refnum<k21>, "error out"=w244:errorcluster)  [unwired: 9 in, 1 out]
          n144 = local write "Digital Waveform Graph"(w187) -> ()
          n145 = local write "Digitaler output"(w187) -> ()
          n146 = call <vilib>:"DAQmx Start Task.vi"("task/channels in"=w245, "error in"=w244) -> ("task out"=w249:refnum<k21>, "error out"=w248:errorcluster)  [unwired: 12 in]
          n147 = flat-sequence {
            tunnel: [w334] -> w256
            tunnel: [w333] -> w255
            tunnel: w252 -> [w332]
            tunnel: w251 -> [w331]
            tunnel: [w330] -> w238
            tunnel: w249 -> [w330]
            tunnel: [w329] -> w237
            tunnel: w248 -> [w329]
            tunnel: [w328] -> w177
            frame #0 {
              n148 = call <vilib>:"DAQmx Start Task.vi"("task/channels in"=w331, "error in"=w332) -> ("task out"=w334:refnum<k21>, "error out"=w333:errorcluster)  [unwired: 12 in]
              n149 = Tick Count (ms)() -> (millisecond timer value=w328:u32)
            }
          }
          n150 = disable-structure shown="Aktiviert" {
            disable-tunnel: w256 -> [w306 _]
            disable-tunnel: w255 -> [w305 _]
            disable-tunnel: [w304 _] -> w181
            disable-tunnel: [w303 _] -> w182
            disable-tunnel: w238 -> [w302 _]
            disable-tunnel: w237 -> [w301 _]
            disable-tunnel: [w300 _] -> w236
            disable-tunnel: [w299 _] -> w176
            disable-tunnel: w177 -> [w298 _]
            disable-tunnel: w169 -> [w297 _]
            frame Enabled {
              n151 = while {
                shift-right: [w324] -> w303
                shift-left: w306 -> [w326]
                shift-right: [w323] -> w304
                shift-left: w305 -> [w325]
                tunnel: w302 -> [w322]
                tunnel: w301 -> [w321]
                tunnel: [w322] -> w300
                tunnel: [w321] -> w299
                tunnel: [w315] -> _
                tunnel: w298 -> [w315]
                tunnel: w297 -> [w312]
                stop <- w317 stop-if-true
                n152 = Tick Count (ms)() -> (millisecond timer value=w313:u32)
                n153 = local read "Stop Boolesch"() -> (w318:bool)
                n154 = Wait (ms)(milliseconds to wait=u32 2 ("Zu wartende ms")) -> ()  [unwired: 1 out]
                n155 = Subtract(x=w313, y=w315) -> (x-y=w308:u32)
                n156 = Subtract(x=w313, y=w312) -> (x-y=w310:u32)
                n157 = call <vilib>:"DAQmx Is Task Done.vi"("task/channels in"=w326, "error in"=w325) -> ("task out"=w324:refnum<k21>, "task done?"=w316:bool, "error out"=w323:errorcluster)  [unwired: 11 in]
                n158 = Unbundle By Name(w323) -> ("status"=w319:bool)
                n159 = Divide(x=w308, y=u32 1000 ("x")) -> (x/y=→"Trial elapsed time":dbl)
                n160 = Divide(x=w310, y=u32 1000 ("x")) -> (x/y=→"Total elapsed time":dbl)
                n161 = Or(x=w319, y=w318) -> (x .or. y?=w327:bool)
                n162 = Or(x=w316, y=w327) -> (x .or. y?=w317:bool)
              }
            }
            frame Disabled {
            }
          }
          n163 = disable-structure shown="Aktiviert" {
            disable-tunnel: w236 -> [w262 _]
            disable-tunnel: [w261 _] -> w180
            disable-tunnel: w176 -> [w260 _]
            disable-tunnel: [w259 _] -> w175
            frame Enabled {
              n164 = call <vilib>:"DAQmx Wait Until Done.vi"("task/channels in"=w262, "error in"=w260) -> ("task out"=w261:refnum<k21>, "error out"=w259:errorcluster)  [unwired: 12 in]
            }
            frame Disabled {
            }
          }
          n165 = flat-sequence {
            tunnel: w182 -> [w281]
            tunnel: w181 -> [w280]
            tunnel: w180 -> [w279]
            tunnel: w175 -> [w278]
            tunnel: w169 -> [w284]
            frame #0 {
              n166 = call <vilib>:"DAQmx Clear Task.vi"("task in"=w281, "error in"=w280) -> ("error out"=w282:errorcluster)  [unwired: 13 in]
              n167 = call <vilib>:"DAQmx Clear Task.vi"("task in"=w279, "error in"=w278) -> ("error out"=w283:errorcluster)  [unwired: 13 in]
              n168 = Merge Errors(w282, w283) -> ()  [unwired: 1 out]
            }
            frame #1 {
              n169 = Tick Count (ms)() -> (millisecond timer value=w285:u32)
              n170 = for {
                N: "Time between trials" -> [_]
                tunnel: w285 -> [w295]
                tunnel: w284 -> [w290]
                stop <- w288 stop-if-true
                w292 = u32 1000 ("Zu wartende ms")
                n171 = Tick Count (ms)() -> (millisecond timer value=w289:u32)
                n172 = Subtract(x=w289, y=w295) -> (x-y=w296:u32)
                n173 = Subtract(x=w289, y=w290) -> (x-y=w293:u32)
                n174 = local read "Stop Boolesch"() -> (w288:bool)
                n175 = Divide(x=w296, y=w292) -> (x/y=→"Pause elapsed time":dbl)
                n176 = Divide(x=w293, y=w292) -> (x/y=w291:dbl)
                n177 = local write "Total elapsed time"(w291) -> ()
                n178 = Wait (ms)(milliseconds to wait=w292) -> ()  [unwired: 1 out]
              }
              "In between trials" <- TRUE ("In between trials")
            }
          }
          n179 = local read "Stop Boolesch"() -> (w183:bool)
          "Current Valve" <- w173
          "Current list index" <- w179
        }
        n180 = local write "Experiment running"(TRUE ("Experiment running")) -> ()
        "State" <- w165
      }
      frame "Stop" {
        n181 = local write "State"(w335) -> ()
        n182 = flat-sequence {
          frame #0 {
            # "Stop-all to zero"
            # "all lines also trigger line"
            n183 = call-poly <vilib>:"DAQmx Write.vi"("task/channels in"="/Dev2/port0/line17:25" ("string"), "data"=bool[] [FALSE, FALSE, FALSE, FALSE, FALSE, FALSE, FALSE, FALSE, FALSE]) -> ("task out"=w343:refnum<k21>, "error out"=w338:errorcluster)  [unwired: 11 in, 1 out]
            n184 = call <vilib>:"DAQmx Start Task.vi"("task/channels in"=w343, "error in"=w338) -> ("task out"=w342:refnum<k21>, "error out"=w340:errorcluster)  [unwired: 12 in]
            n185 = call <vilib>:"DAQmx Wait Until Done.vi"("task/channels in"=w342, "error in"=w340) -> ("task out"=w341:refnum<k21>, "error out"=w339:errorcluster)  [unwired: 12 in]
            n186 = call <vilib>:"DAQmx Clear Task.vi"("task in"=w341, "error in"=w339) -> ()  [unwired: 13 in, 1 out]
          }
          frame #1 {
            w349 = T2."Enabled" ("Deaktiviert")
            n187 = property on="Select experiment" class="TabCtl (strict)"() -> ("Pages"=w348:refnum<vi>[])  [unwired: 2 in, 2 out]
            n188 = property on="Valve order list" class="Arr (strict)"("DisabledEnum"=T2."Enabled" ("Deaktiviert")) -> ()  [unwired: 2 in, 2 out]
            n189 = for {
              tunnel: w348 -> [w350] mode=indexing
              n190 = property class="Page"(reference=w350, "PageEnb"=T3."Page Enabled" ("Aktiv-Status der Seite")) -> ()  [unwired: 1 in, 2 out]
            }
            n191 = property on="Start trial series" class="Bool"("DisabledEnum"=w349) -> ()  [unwired: 2 in, 2 out]
            n192 = property on="Start single trial" class="Bool"("DisabledEnum"=w349) -> ()  [unwired: 2 in, 2 out]
            "Experiment running" <- FALSE ("Experiment running")
          }
        }
        n193 = local read "Stop Boolesch"() -> (w337:bool)
      }
    }
  }
  n194 = while {
    tunnel: w4 -> [w353]
    stop <- w352 stop-if-true
    n195 = event shown="[2] \"Stopp\": Value Change" {
      selector: _ -> [_ _ _ _]
      dyn-events: _ -> [_ _ _ _]
      timeout: _ -> [_ _ _ _]
      tunnel: w353 -> [_ w354 w363 w369]
      event Timeout {
        n196 = event-data() -> ()  [unwired: 1 in, 3 out]
      }
      event "Start single trial": Value Change {
        n197 = event-data() -> ()  [unwired: 1 in, 6 out]
        n198 = case shown="True" "Start single trial" {
          tunnel: w354 -> [_ w362]
          frame False {
          }
          frame True {
            n199 = property on="Start single trial" class="Bool"("DisabledEnum"=T2."Disabled and Grayed Out" ("Deaktiviert")) -> ()  [unwired: 2 in, 2 out]
            n200 = Enqueue Element(queue=w362, element=StatesEnum."Start Trial" ("Enum")) -> ()  [unwired: 2 in, 3 out]
            n201 = property on="Select experiment" class="TabCtl (strict)"() -> ("Pages"=w358:refnum<vi>[])  [unwired: 2 in, 2 out]
            n202 = Index Array(array=w358, index=1 ("Index")) -> (element=w359:refnum<vi>)
            n203 = property class="Page"(reference=w359, "PageEnb"=T3."Page Disabled & Grayed" ("Aktiv-Status der Seite")) -> ()  [unwired: 1 in, 2 out]
          }
        }
      }
      event "Stopp": Value Change {
        n204 = event-data() -> ()  [unwired: 1 in, 6 out]
        n205 = case shown="True" "Stopp" {
          tunnel: w363 -> [_ w367]
          frame False {
          }
          frame True {
            n206 = Enqueue Element(queue=w367, element=StatesEnum."Stop" ("Enum")) -> ()  [unwired: 2 in, 3 out]
            "Stop Boolesch" <- TRUE ("Stop Boolesch")
          }
        }
      }
      event "Start trial series": Value Change {
        n207 = event-data() -> ()  [unwired: 1 in, 6 out]
        n208 = case shown="True" "Start trial series" {
          tunnel: w369 -> [_ w376]
          frame False {
          }
          frame True {
            n209 = property on="Start trial series" class="Bool"("DisabledEnum"=T2."Disabled and Grayed Out" ("Deaktiviert")) -> ()  [unwired: 2 in, 2 out]
            n210 = Enqueue Element(queue=w376, element=StatesEnum."Start trial series" ("Enum")) -> ()  [unwired: 2 in, 3 out]
            n211 = property on="Select experiment" class="TabCtl (strict)"() -> ("Pages"=w372:refnum<vi>[])  [unwired: 2 in, 2 out]
            n212 = Index Array(array=w372, index=0 ("Index")) -> (element=w373:refnum<vi>)
            n213 = property class="Page"(reference=w373, "PageEnb"=T3."Page Disabled & Grayed" ("Aktiv-Status der Seite")) -> ()  [unwired: 1 in, 2 out]
          }
        }
      }
    }
    n214 = local read "Stop Boolesch"() -> (w352:bool)
  }
  n215 = Release Queue(queue=w3) -> ()  [unwired: 2 in, 3 out]
